vi "ExecuteGrSimTest.vi"(4 "Number of Points":i32, 6 "Replace Robots":bool, 7 "IA State Input":T3, 8 "Test Mode On":bool, 9 "reset":bool, 10 "id":i32, 11 "RandomAllyPoints":dbl[][](array[numeric])) -> (1 "kick num":i32, 2 "Replace active":bool, 3 "grSim replacement":cluster{"robots":T1[], "ball":T2}={"robots"=[{"x"=0.0, "y"=-450.0, "dir"=0.0, "yellowteam"=FALSE, "id"=0}, {"x"=0.0, "y"=-270.0, "dir"=0.0, "yellowteam"=FALSE, "id"=1}, {"x"=0.0, "y"=-90.0, "dir"=0.0, "yellowteam"=FALSE, "id"=2}, {"x"=0.0, "y"=90.0, "dir"=0.0, "yellowteam"=FALSE, "id"=3}, {"x"=0.0, "y"=270.0, "dir"=0.0, "yellowteam"=FALSE, "id"=4}, {"x"=0.0, "y"=450.0, "dir"=0.0, "yellowteam"=FALSE, "id"=5}], "ball"={"x"=0.0, "y"=0.0, "vx"=0.0, "vy"=0.0}})   [LabVIEW 2017]
uses:
  Core/AI Input.ctl
  Core/AI Robot.ctl
  Intel/Functions Enum.ctl
  Intel/AttackerStates.ctl
  Path Planning/RRT/PathDests.ctl
  Path Planning/RRT/PathDest.ctl
  Core/AI Ball.ctl
  Core/Field Size.ctl
  Core/AI Judge.ctl
  Intel/Command Enum.ctl
  Util/Events/Events.ctl
  grSim RobotReplacement.ctl
  grSim_BallReplacement.ctl
panel:
  in  "Time":enum16{"Azul", "Amarelo"}(ring) caption="Enum"
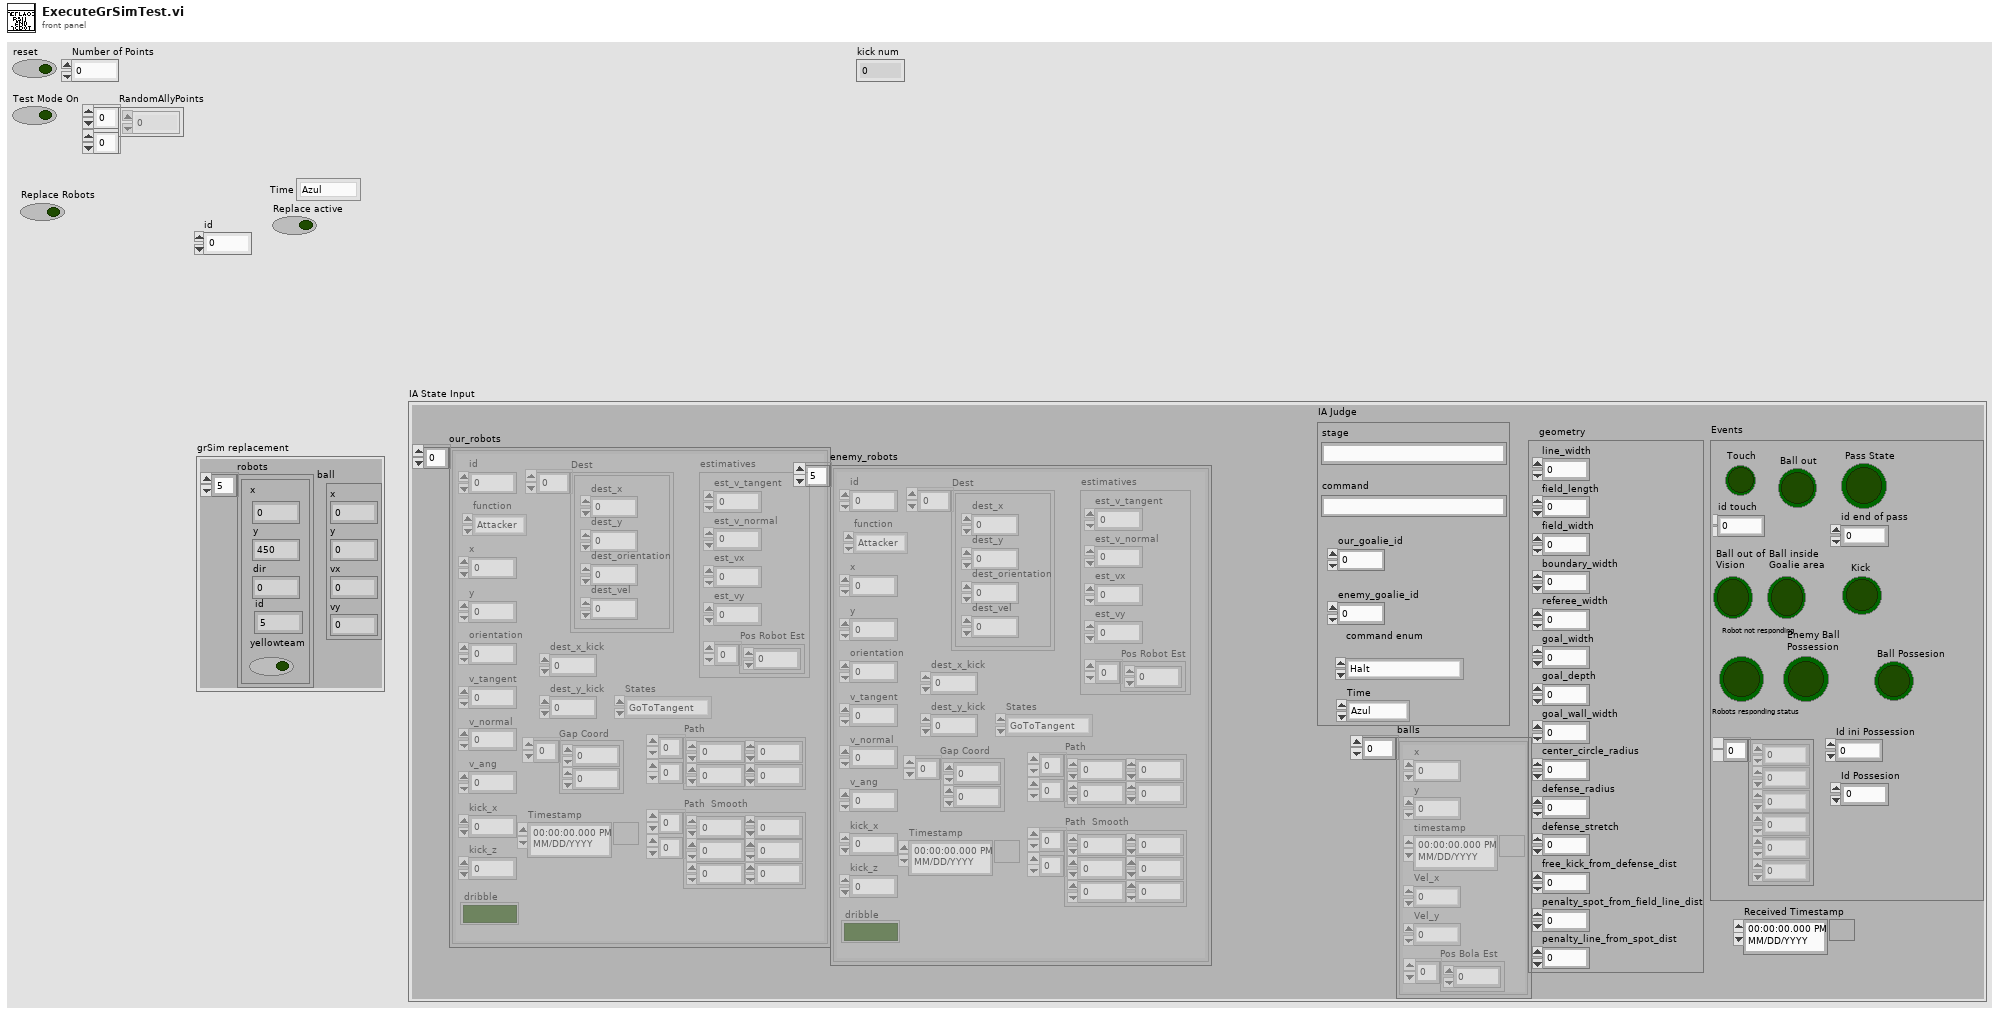
[diagram p1: front panel]
types:
  T1 = typedef "grSim RobotReplacement.ctl" = cluster{"x":dbl, "y":dbl, "dir":dbl, "yellowteam":bool, "id":u32}
  T2 = typedef "grSim_BallReplacement.ctl" = cluster{"x":dbl, "y":dbl, "vx":dbl, "vy":dbl}
  T3 = typedef "AI Input.ctl" = cluster{"our_robots":T4[], "enemy_robots":T4[], "balls":T9[], "geometry":T10, "IA Judge":T11, "Received Timestamp":timestamp, "Events":T13}
  T4 = typedef "AI Robot.ctl" = cluster{"id":u32, "function":T5, "x":dbl, "y":dbl, "orientation":dbl, "v_tangent":dbl, "v_normal":dbl, "v_ang":dbl, "kick_x":dbl, "kick_z":dbl, "dribble":bool, "Timestamp":timestamp, "estimatives":cluster{"est_v_tangent":dbl, "est_v_normal":dbl, "est_vx":dbl, "est_vy":dbl, "Pos Robot Est":dbl[]}, "dest_x_kick":dbl, "dest_y_kick":dbl, "Gap Coord":dbl[], "States":T6, "Path ":dbl[][], "Path  Smooth":dbl[][], "Dest":T7}
  T5 = typedef "Functions Enum.ctl" = enum16{"Attacker", "Goalie", "Defender", "Striker", "Goto 0", "Dummy", "Kicker", "ZigZag"}
  T6 = typedef "AttackerStates.ctl" = enum16{"Pass", "GoToTangent", "BallGetting", "GoToKick", ""}
  T7 = typedef "PathDests.ctl" = T8[]
  T8 = typedef "PathDest.ctl" = cluster{"dest_x":dbl, "dest_y":dbl, "dest_orientation":dbl, "dest_vel":dbl}
  T9 = typedef "AI Ball.ctl" = cluster{"x":dbl, "y":dbl, "timestamp":timestamp, "Vel_x":dbl, "Vel_y":dbl, "Pos Bola Est":dbl[]}
  T10 = typedef "Field Size.ctl" = cluster{"line_width":u32, "field_length":u32, "field_width":u32, "boundary_width":u32, "referee_width":u32, "goal_width":u32, "goal_depth":u32, "goal_wall_width":u32, "center_circle_radius":u32, "defense_radius":u32, "defense_stretch":u32, "free_kick_from_defense_dist":u32, "penalty_spot_from_field_line_dist":u32, "penalty_line_from_spot_dist":u32}
  T11 = typedef "AI Judge.ctl" = cluster{"stage":string, "command":string, "our_goalie_id":dbl, "enemy_goalie_id":dbl, "command enum":T12, "Time":enum16{"Azul", "Amarelo"}}
  T12 = typedef "Command Enum.ctl" = enum16{"Halt", "Stop", "Force Start", "PKA Normal Start", "Prepare Kickoff Ally", "PKE Normal Start", "Prepare Kickoff Enemy", "Prepare Penalty Ally", "PPA Normal Start", "Prepare Penalty Enemy", "PPE Normal Start", "Direct Free Enemy", "Direct Free Ally", "Indirect Free Enemy", "Indirect Free Ally", "Timeout Enemy", "Timeout Ally", "Goal Enemy", "Goal Ally", "Ball Placement Enemy", "Ball Placement Ally", "Normal Half Time", "Extra Time Break", "Extra Half Time", "None", "Post Game"}
  T13 = typedef "Events.ctl" = cluster{"Touch":bool, "Ball out":bool, "id touch":dbl, "Ball out of \nVision":bool, "Ball inside \nGoalie area":bool, "Robot not responding":bool, "Robots responding status":dbl[], "Enemy Ball \nPossession":bool, "Pass State":bool, "id end of pass":dbl, "Kick":bool, "Id ini Possession":dbl, "Ball Possesion":bool, "Id Possesion":dbl}
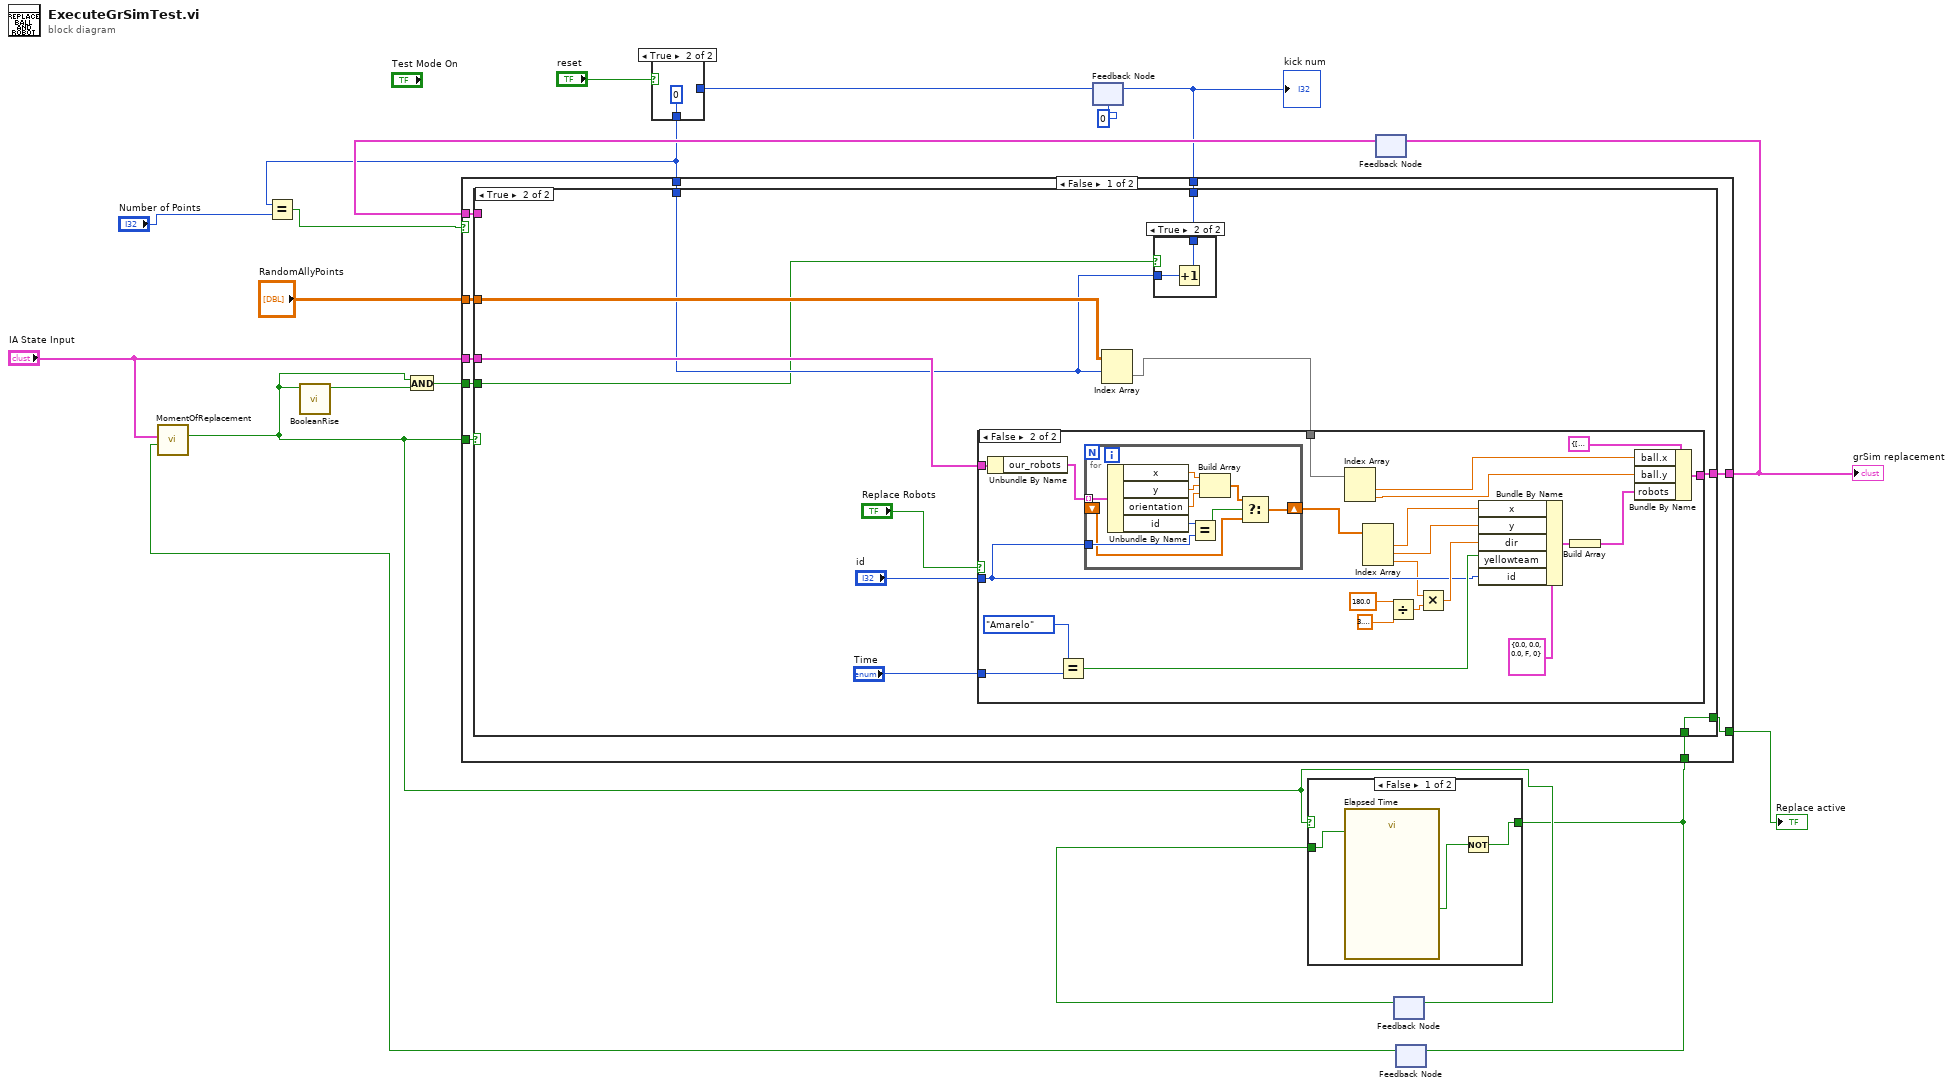
[diagram p0: block diagram]
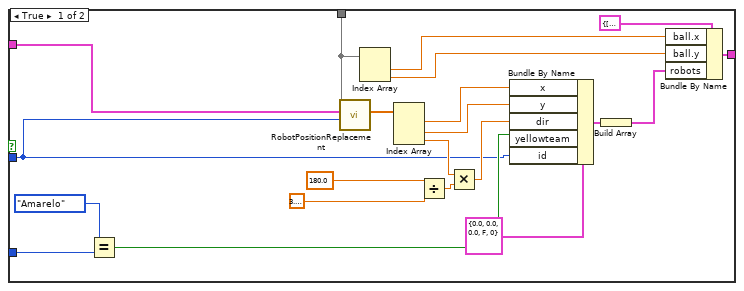
[diagram p4: hidden frame]
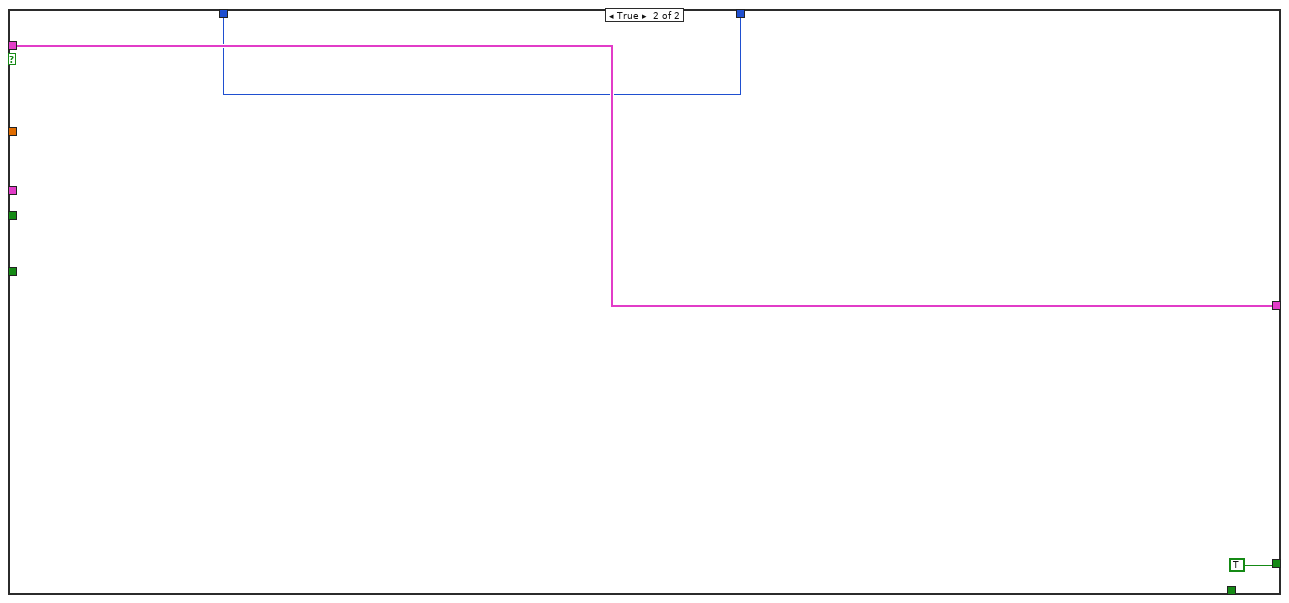
[diagram p5: hidden frame]
diagram:
  n1 = feedback #1(0) -> (w7:i32)
  n2 = case shown="True" "reset" {
    tunnel: w7 -> [w19 _]
    tunnel: [w19 0] -> w4
    frame False {
    }
    frame True {
    }
  }
  n3 = Equal?(x=w4, y="Number of Points") -> (x = y?=w3:bool)
  n4 = feedback #2() -> (w18:cluster{"robots":T1[], "ball":T2})  [unwired: 1 in]
  n5 = feedback #3() -> (w17:bool)  [unwired: 1 in]
  n6 = feedback #4() -> (w14:bool)  [unwired: 1 in]
  n7 = call "MomentOfReplacement.vi"("Replace active"=w14, "IA State Input"="IA State Input") -> ("Time to replace?"=w8:bool)  [unwired: 9 in]
  n8 = call "BooleanRise.vi"("Test Mode On"=w8) -> ("Boolean"=w9:bool)  [unwired: 10 in]
  n9 = And(x=w8, y=w9) -> (x .and. y?=w10:bool)
  n10 = case shown="False" w8 {
    selector: w8 -> [_ w24]
    tunnel: [w23 w24] -> w2
    tunnel: w17 -> [w21 _]
    frame False {
      n11 = call "Elapsed Time"("Reset"=w21) -> ("Time has Elapsed"=w22:bool)  [unwired: 11 in, 7 out]
      n12 = Not(x=w22) -> (.not. x?=w23:bool)
    }
    frame True {
    }
  }
  n13 = case shown="False" w3 {
    tunnel: w18 -> [w34 w106]
    tunnel: [w33 w106] -> w16
    tunnel: "IA State Input" -> [w32 _]
    tunnel: "RandomAllyPoints" -> [w31 _]
    tunnel: [w30 w105] -> w11
    tunnel: w10 -> [w29 _]
    tunnel: w8 -> [w28 _]
    tunnel: w4 -> [w27 w105]
    tunnel: w2 -> [w25 _]
    tunnel: [w26 TRUE] -> w1
    frame False {
      n14 = case shown="True" w28 {
        tunnel: [w37 w48] -> w33
        tunnel: w32 -> [_ w45]
        tunnel: w34 -> [w37 _]
        tunnel: w31 -> [_ w44]
        tunnel: w27 -> [w36 w41]
        tunnel: [w36 w40] -> w30
        tunnel: w29 -> [_ w39]
        tunnel: [w35 w38] -> w26
        tunnel: w25 -> [w35 w38]
        frame False {
        }
        frame True {
          n15 = Index Array(array=w44, index (row)=w41) -> (element=w47:dbl[])  [unwired: 1 in]
          n16 = case shown="False" "Replace Robots" {
            tunnel: [w72 w94] -> w48
            tunnel: w47 -> [w55 w76]
            tunnel: "Time" -> [w68 w90]
            tunnel: w45 -> [w63 w83]
            tunnel: "id" -> [w56 w81]
            frame True {
              n17 = Equal?(x=enum16{"Azul", "Amarelo"}."Amarelo", y=w68) -> (x = y?=w66:bool)
              n18 = call "RobotPositionReplacement.vi"("id"=w56, "IA State Input"=w63, "Position Ball"=w55) -> ("Position Robot"=w65:dbl[])  [unwired: 6 in]
              n19 = Index Array(array=w55) -> (element #1=w54:dbl, element #2=w53:dbl)  [unwired: 2 in]
              n20 = Index Array(array=w65) -> (element #1=w64:dbl, element #2=w62:dbl, element #3=w57:dbl)  [unwired: 3 in]
              n21 = Divide(x=180.0, y=3.141592653589793) -> (x/y=w60:dbl)
              n22 = Multiply(x=w57, y=w60) -> (x*y=w61:dbl)
              n23 = Bundle By Name(cluster=T1 {"x"=0.0, "y"=0.0, "dir"=0.0, "yellowteam"=FALSE, "id"=0} ("element"), "x"=w64, "y"=w62, "dir"=w61, "yellowteam"=w66, "id"=w56) -> (w70:T1)
              n24 = Build Array(w70) -> (w69:T1[])
              n25 = Bundle By Name(cluster=cluster{"robots":T1[], "ball":T2} {"robots"=[{"x"=0.0, "y"=-450.0, "dir"=0.0, "yellowteam"=FALSE, "id"=0}, {"x"=0.0, "y"=-270.0, "dir"=0.0, "yellowteam"=FALSE, "id"=1}, {"x"=0.0, "y"=-90.0, "dir"=0.0, "yellowteam"=FALSE, "id"=2}, {"x"=0.0, "y"=90.0, "dir"=0.0, "yellowteam"=FALSE, "id"=3}, {"x"=0.0, "y"=270.0, "dir"=0.0, "yellowteam"=FALSE, "id"=4}, {"x"=0.0, "y"=450.0, "dir"=0.0, "yellowteam"=FALSE, "id"=5}], "ball"={"x"=0.0, "y"=0.0, "vx"=0.0, "vy"=0.0}} ("grSim replacement"), "ball.x"=w54, "ball.y"=w53, "robots"=w69) -> (w72:cluster{"robots":T1[], "ball":T2})
            }
            frame False {
              n26 = Unbundle By Name(w83) -> ("our_robots"=w82:T4[])
              n27 = Equal?(x=enum16{"Azul", "Amarelo"}."Amarelo", y=w90) -> (x = y?=w88:bool)
              n28 = for {
                tunnel: w82 -> [w104] mode=indexing
                tunnel: w81 -> [w102]
                shift-right: [w96] -> w80
                shift-left: _ -> [w95]
                n29 = Unbundle By Name(w104) -> ("x"=w101:dbl, "y"=w100:dbl, "orientation"=w99:dbl, "id"=w103:u32)
                n30 = Equal?(x=w103, y=w102) -> (x = y?=w98:bool)
                n31 = Build Array(w101, w100, w99) -> (w97:dbl[])
                n32 = Select(t=w97, s=w98, f=w95) -> (s? t:f=w96:dbl[])
              }
              n33 = Index Array(array=w76) -> (element #1=w75:dbl, element #2=w74:dbl)  [unwired: 2 in]
              n34 = Index Array(array=w80) -> (element #1=w79:dbl, element #2=w77:dbl, element #3=w78:dbl)  [unwired: 3 in]
              n35 = Divide(x=180.0, y=3.141592653589793) -> (x/y=w86:dbl)
              n36 = Multiply(x=w78, y=w86) -> (x*y=w87:dbl)
              n37 = Bundle By Name(cluster=T1 {"x"=0.0, "y"=0.0, "dir"=0.0, "yellowteam"=FALSE, "id"=0} ("element"), "x"=w79, "y"=w77, "dir"=w87, "yellowteam"=w88, "id"=w81) -> (w92:T1)
              n38 = Build Array(w92) -> (w91:T1[])
              n39 = Bundle By Name(cluster=cluster{"robots":T1[], "ball":T2} {"robots"=[{"x"=0.0, "y"=-450.0, "dir"=0.0, "yellowteam"=FALSE, "id"=0}, {"x"=0.0, "y"=-270.0, "dir"=0.0, "yellowteam"=FALSE, "id"=1}, {"x"=0.0, "y"=-90.0, "dir"=0.0, "yellowteam"=FALSE, "id"=2}, {"x"=0.0, "y"=90.0, "dir"=0.0, "yellowteam"=FALSE, "id"=3}, {"x"=0.0, "y"=270.0, "dir"=0.0, "yellowteam"=FALSE, "id"=4}, {"x"=0.0, "y"=450.0, "dir"=0.0, "yellowteam"=FALSE, "id"=5}], "ball"={"x"=0.0, "y"=0.0, "vx"=0.0, "vy"=0.0}} ("grSim replacement"), "ball.x"=w75, "ball.y"=w74, "robots"=w91) -> (w94:cluster{"robots":T1[], "ball":T2})
            }
          }
          n40 = case shown="True" w39 {
            tunnel: w41 -> [w49 w51]
            tunnel: [w49 w50] -> w40
            frame False {
            }
            frame True {
              n41 = Increment(x=w51) -> (x+1=w50:i32)
            }
          }
        }
      }
    }
    frame True {
    }
  }
  "grSim replacement" <- w16
  "Replace active" <- w1
  "kick num" <- w11
  n42 = feedback-in #1(w11) -> ()
  n43 = feedback-in #2(w16) -> ()
  n44 = feedback-in #3(w8) -> ()
  n45 = feedback-in #4(w2) -> ()
